vi "Untitled 1 (SubVI).vi"(4 "color(black)":u32(colorbox), 6 "# Rows":i8, 7 "dimensions":cluster{"Width":i32, "Height":i32}, 8 "Row":i32, 9 "# Columns":i8, 10 "Column":i32, 11 "image":picture) -> (3 "new picture":picture)   [LabVIEW 2012]
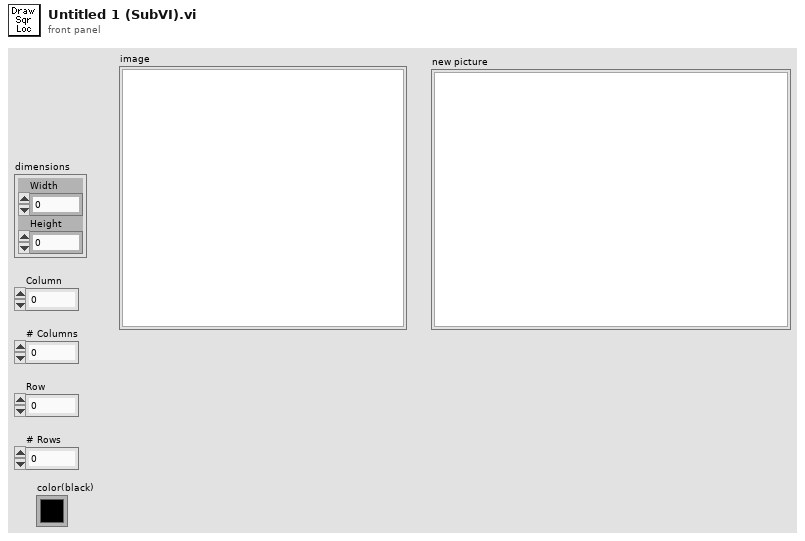
[diagram p1: front panel]
types:
  T1 = cluster{"Width":i16, "Style":enum32{"Solid", "Dash", "Dot", "DashDot", "DashDotDot"}}
  T2 = cluster{"left":i16, "top":i16, "right":i16, "bottom":i16}
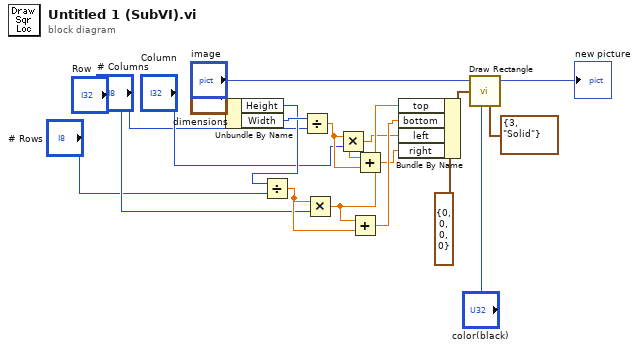
[diagram p0: block diagram]
diagram:
  n1 = Unbundle By Name("dimensions") -> ("Height"=w12:i32, "Width"=w15:i32)
  n2 = Divide(x=w12, y="# Rows") -> (x/y=w17:dbl)
  n3 = Divide(x=w15, y="# Columns") -> (x/y=w16:dbl)
  n4 = Multiply(x=w17, y="Row") -> (x*y=w18:dbl)
  n5 = Multiply(x=w16, y="Column") -> (x*y=w10:dbl)
  n6 = Add(x=w18, y=w17) -> (x+y=w19:dbl)
  n7 = Add(x=w10, y=w16) -> (x+y=w11:dbl)
  n8 = Bundle By Name(cluster=T2 {"left"=0, "top"=0, "right"=0, "bottom"=0} ("rect"), "top"=w18, "bottom"=w19, "left"=w10, "right"=w11) -> (w4:T2)
  n9 = call <vilib>:"Draw Rectangle.vi"("picture"="image", "rect"=w4, "color(black)"="color(black)", "pen"=T1 {"Width"=3, "Style"=enum."Solid"}) -> ("new picture"=→"new picture":picture)  [unwired: 5 in]
